vi "Subtask1A (1).vi"() -> ()   [LabVIEW 2016, in "Team234_Project5.lvrbt"]
uses:
  Team234_Project5.lvrbt
  <vilib>/NXT/Block Support/NXT_OutputPort.ctl
  <vilib>/NXT/Subs/LVHSConnector.ctl
  <vilib>/NXT/LegoClasses/BrickReference/BrickReference.lvclass
  <vilib>/NXT/NXTIO Xnodes/NXTIONodeSubVIs/NXTMoveMotors.vi
  <vilib>/NXT/Dual Mode Library/Waits/Wait_Num.vi
  <vilib>/NXT/NXTIO Xnodes/NXTIONodeSubVIs/NXTStopMotors.vi
  <vilib>/NXT/NXTIO Xnodes/NXTIOXNode/NXTIO.xnode
panel:
  in  "Time (1 sec) 5":sgl=1.0
  in  "Loop Executions":i32
  in  "Time (1 sec) 4":sgl=1.0
  in  "Large Motor B Phase 2":i8=75
  in  "Large Motor A Phase 2":i8=75
  in  "Large Motor A":i8=75
  in  "NXT/EV3 6":T1
  in  "Port Selection Motor A":T2=7 items=["Port A", "Port B", "Port C", "Port D"]
  in  "NXT/EV3 2":T1
  in  "Port Selection Motor B":T2=7 items=["Port A", "Port B", "Port C", "Port D"]
  in  "Large Motor B":i8=75
  # "Timers for execution"
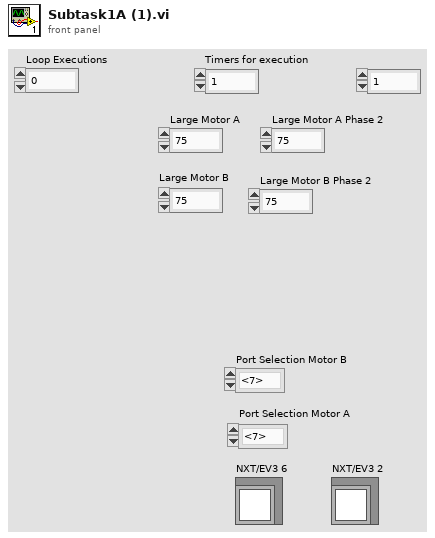
[diagram p1: front panel]
types:
  T1 = typedef "LVHSConnector.ctl" = refnum<class "BrickReference.lvclass">
  T2 = typedef "NXT_OutputPort.ctl" = u8
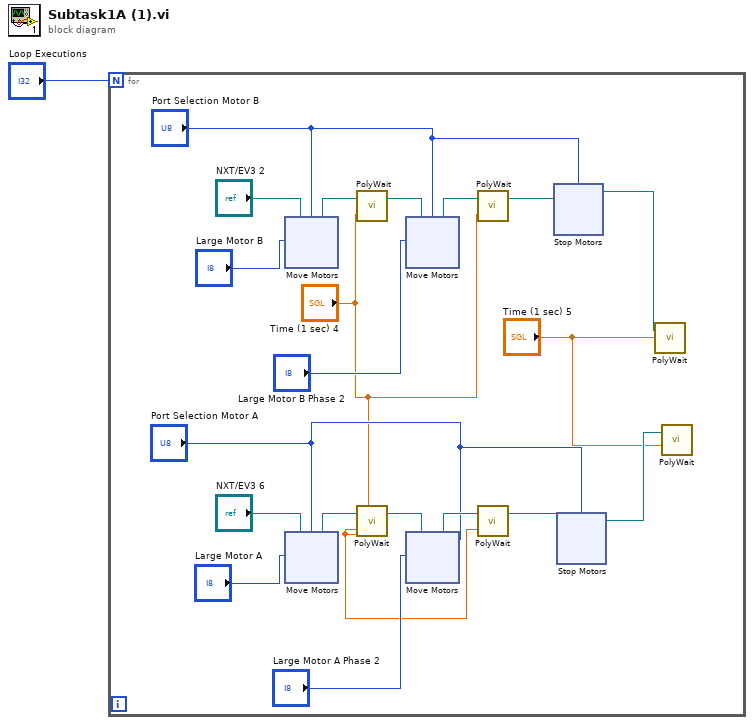
[diagram p0: block diagram]
diagram:
  n1 = for {
    N: "Loop Executions" -> [_]
    n2 = xnode "Move Motors"("Power/Speed 1"="Large Motor B", "Motors"="Port Selection Motor B", "NXT/EV3"="NXT/EV3 2") -> ("NXT/EV3"=w14:T1)
    n3 = xnode "Move Motors"("Power/Speed 1"="Large Motor A", "Motors"="Port Selection Motor A", "NXT/EV3"="NXT/EV3 6") -> ("NXT/EV3"=w18:T1)
    n4 = call-poly <vilib>:"PolyWait.vi"("Time (1 sec)"="Time (1 sec) 4", "NXT/EV3"=w14) -> ("NXT/EV3"=w13:T1)  [unwired: 2 in]
    n5 = call-poly <vilib>:"PolyWait.vi"("Time (1 sec)"="Time (1 sec) 4", "NXT/EV3"=w18) -> ("NXT/EV3"=w17:T1)  [unwired: 2 in]
    n6 = xnode "Move Motors"("Power/Speed 1"="Large Motor B Phase 2", "Motors"="Port Selection Motor B", "NXT/EV3"=w13) -> ("NXT/EV3"=w11:T1)
    n7 = xnode "Move Motors"("Power/Speed 1"="Large Motor A Phase 2", "Motors"="Port Selection Motor A", "NXT/EV3"=w17) -> ("NXT/EV3"=w12:T1)
    n8 = call-poly <vilib>:"PolyWait.vi"("Time (1 sec)"="Time (1 sec) 4", "NXT/EV3"=w11) -> ("NXT/EV3"=w9:T1)  [unwired: 2 in]
    n9 = call-poly <vilib>:"PolyWait.vi"("Time (1 sec)"="Time (1 sec) 4", "NXT/EV3"=w12) -> ("NXT/EV3"=w6:T1)  [unwired: 2 in]
    n10 = xnode "Stop Motors"("Motors"="Port Selection Motor B", "NXT/EV3"=w9) -> ("NXT/EV3"=w5:T1)
    n11 = xnode "Stop Motors"("Motors"="Port Selection Motor A", "NXT/EV3"=w6) -> ("NXT/EV3"=w4:T1)
    n12 = call-poly <vilib>:"PolyWait.vi"("Time (1 sec)"="Time (1 sec) 5", "NXT/EV3"=w5) -> ()  [unwired: 2 in, 1 out]
    n13 = call-poly <vilib>:"PolyWait.vi"("Time (1 sec)"="Time (1 sec) 5", "NXT/EV3"=w4) -> ()  [unwired: 2 in, 1 out]
  }
